vi "Write position(x,y).vi"(8 "error in (no error)":errorcluster, 10 "position(x,y)":dbl[](array[numeric]), 11 "Object in":refnum<class "Object.lvclass">) -> (0 "error out":errorcluster, 3 "Object out":refnum<class "Object.lvclass">)   [LabVIEW 2020, in "Object.lvclass"]
uses:
  Object.lvclass
  Object.lvclass/Object.ctl
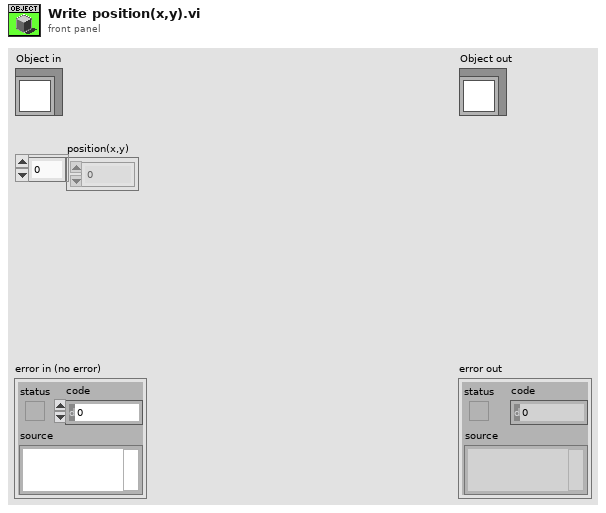
[diagram p1: front panel]
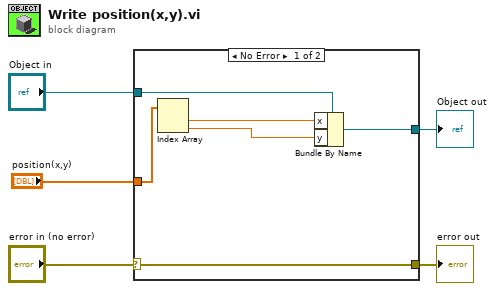
[diagram p0: block diagram]
diagram:
  n1 = case shown="No Error" "error in (no error)" {
    selector: "error in (no error)" -> [w11 w12]
    tunnel: [w11 w12] -> w4
    tunnel: [w9 w13] -> w2
    tunnel: "Object in" -> [w10 w13]
    tunnel: "position(x,y)" -> [w8 _]
    frame No Error {
      n2 = Index Array(array=w8) -> (element #1=w7:dbl, element #2=w6:dbl)  [unwired: 2 in]
      n3 = Bundle By Name(cluster=w10, "x"=w7, "y"=w6) -> (w9:refnum<class "Object.lvclass">)
    }
    frame Error {
    }
  }
  "error out" <- w4
  "Object out" <- w2
